vi "FlashWindow.vi"(8 "error in (no error)":errorcluster, 10 "bInvert? (f)":bool, 11 "hWnd (null)":T1) -> (0 "error out":errorcluster, 2 "Previously Active?":bool, 3 "dup hWnd":T1)   [LabVIEW 2011]
doc: "FlashWindow\nThe FlashWindow function flashes the specified window once, whereas the FlashWindowEx function flashes a specified number of times. \n\nBOOL FlashWindow(\n HWND hWnd, // handle to window to flash\n BOOL bInvert // flash status\n);\n \nParameters\nhWnd \nHandle to the window to be flashed. The window can be either open or minimized (iconic). \nbInvert \nSpecifies whether the window is to be flashed or returned to its original state. The window is flashed from one state to the other if this parameter is TRUE. If it is FALSE, the window is returned to its original state (either active or inactive). When an application is iconic, if this parameter is TRUE, the taskbar window button flashes active/inactive. If it is FALSE, the taskbar window button flashes inactive, meaning that it does not change colors. It flashes, as if it were being redraw, but it does not provide the visual invert clue to the user. \nReturn Values\nThe return value specifies the window's state before the call to the FlashWindow function. If the window was active before the call, the return value is nonzero. \n\nIf the window was not active before the call, the return value is zero. \n\nRemarks\nFlashing a window means changing the appearance of its caption bar as if the window were changing from inactive to active status, or vice versa. (An inactive caption bar changes to an active caption bar; an active caption bar changes to an inactive caption bar.) \n\nTypically, a window is flashed to inform the user that the window requires attention but that it does not currently have the keyboard focus. \n\nThe FlashWindow function flashes the window only once; for repeated flashing, the application should create a system timer."
uses:
  hWnd.ctl
  user32.dll
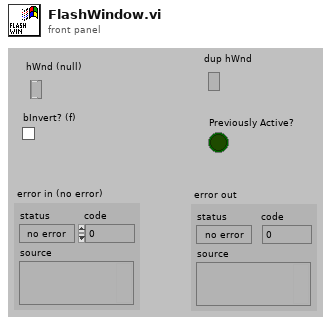
[diagram p1: front panel]
types:
  T1 = typedef "hWnd.ctl" = refnum<k1>
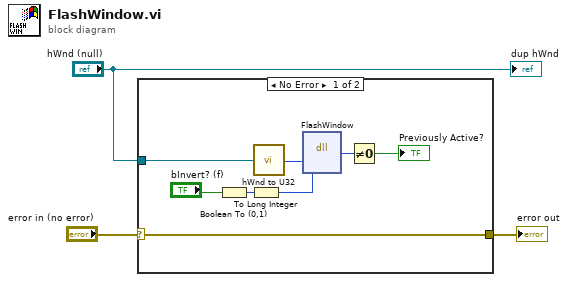
[diagram p0: block diagram]
diagram:
  n1 = case shown="No Error" "error in (no error)" {
    selector: "error in (no error)" -> [w8 w12]
    tunnel: "hWnd (null)" -> [w10 _]
    tunnel: [w8 w12] -> w1
    frame No Error {
      n2 = Boolean To (0,1)(Boolean="bInvert? (f)") -> (0, 1=w5:i16)
      n3 = To Long Integer(number=w5) -> (32bit integer=w4:i32)
      n4 = call "hWnd to U32.vi"("hWnd"=w10) -> ("hWnd"=w11:u32)  [unwired: 4 out]
      n5 = dll-call lib="User32.dll" fn="FlashWindow"("hWnd"=w11, "bInvert"=w4) -> ("active?"=w9:i32)  [unwired: 5 in, 2 out]
      n6 = Not Equal To 0?(x=w9) -> (x != 0?=→"Previously Active?":bool)
    }
    frame Error {
    }
  }
  "error out" <- w1
  "dup hWnd" <- "hWnd (null)"
